vi "IMAQ FPGA Image Transfer to Target.vi"   [LabVIEW 2020, in "NI_VDM_FPGA_Basics.lvlib"]
doc: "Transfers an image from the host processor to the target FPGA via a DMA FIFO."
uses:
  <vilib>/visionFPGA/NI_VDM_FPGA_Basics.lvlib
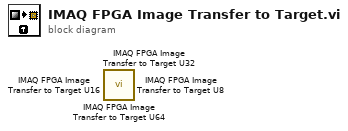
[diagram p0: block diagram]
diagram:
  n1 = call <vilib>:"IMAQ FPGA Image Transfer to Target U64.vi"() -> ()  [unwired: 9 in, 3 out]
  n2 = call <vilib>:"IMAQ FPGA Image Transfer to Target U32.vi"() -> ()  [unwired: 9 in, 3 out]
  n3 = call <vilib>:"IMAQ FPGA Image Transfer to Target U16.vi"() -> ()  [unwired: 9 in, 3 out]
  n4 = call <vilib>:"IMAQ FPGA Image Transfer to Target U8.vi"() -> ()  [unwired: 9 in, 3 out]
